vi "Lidar V5.2 RT Main.vi"() -> ()   [LabVIEW 2015]
uses:
  <vilib>/userdefined/niP2PState.ctl
  LIDAR Globals.vi
  <vilib>/Utility/error.llb/Error Cluster From Error Code.vi
  <vilib>/rvi/errors/niLvFpgaAdjustHostInterfaceError.vi
  <vilib>/rvi/interface/nirviMethod/nirviMethod.xnode
  <vilib>/rvi/interface/nirviReadWriteControl/nirviReadWriteControl.xnode
  <vilib>/rvi/errors/niLvFpgaMergeErrorWithErrorCode.vi
  <resource>/objmgr/PeerToPeerStream.rc
  <vilib>/FPGAPlugInAG/Dynamic/niLvFpga_ReadFifo_Dynamic.vi
  NiFpgaLv.dll
  <vilib>/rvi/interface/Simulation/niFpgaSimulationCallBeginRW.vi
panel:
  out "Frames":i32
  out "Slave Ref":refnum<k20>
  out "Master Ref":refnum<k20>
  out "P2P ref":refnum<k20>
  in  "Init Fpga":bool
  in  "ReadSingleFrame":bool
  out "ExitApp":bool
  out "Elements Remaining 2":u32
  in  "ReadSamples":bool
  out "Data":dbl[](graph)
  in  "stop":bool
  out "State":T1
  out "error out":errorcluster
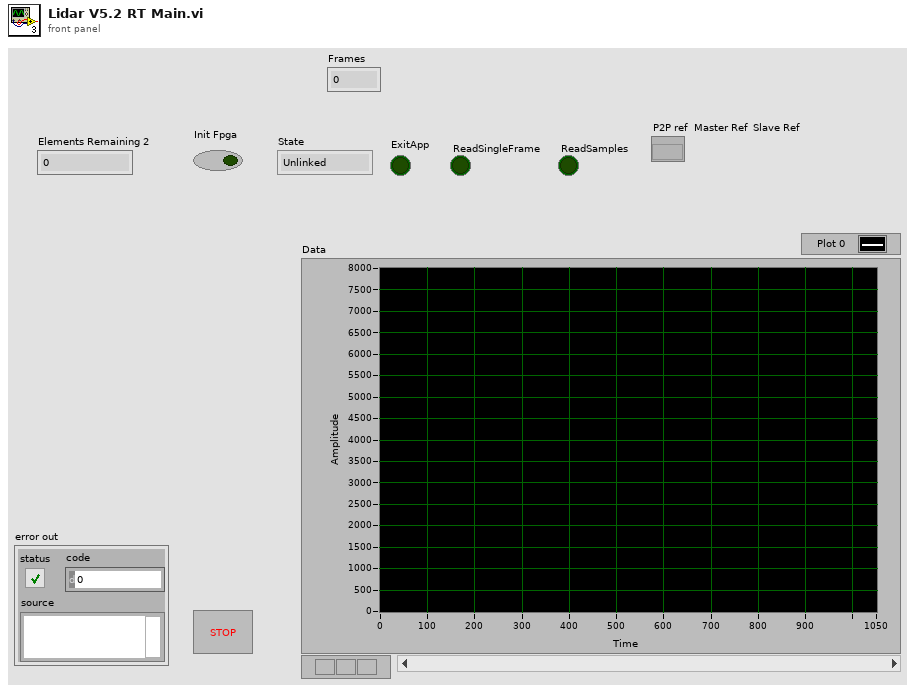
[diagram p1: front panel]
types:
  T1 = typedef "niP2PState.ctl" = enum32{"Unlinked", "Disabled", "Enabled", "Flushing"}
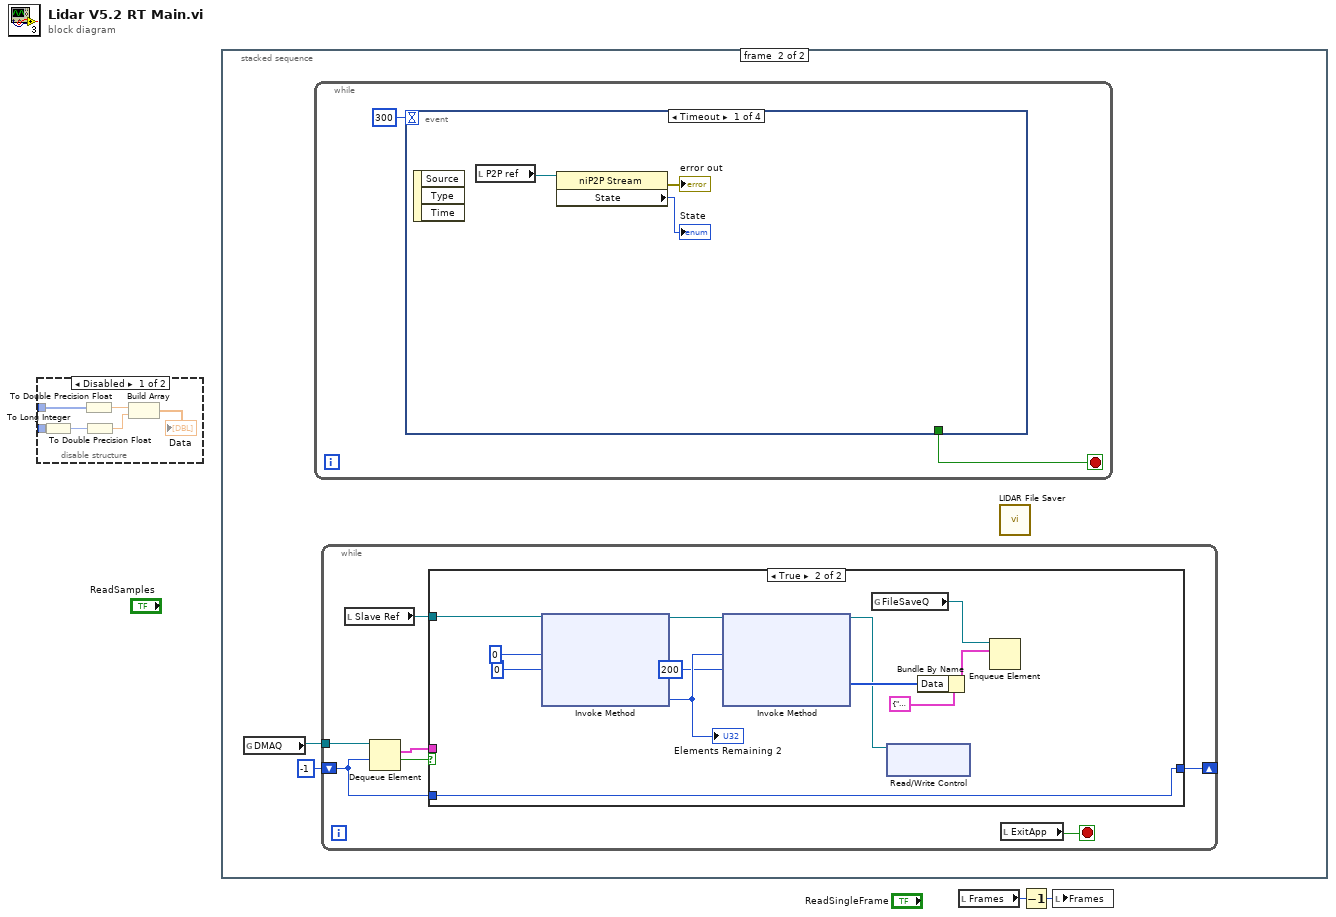
[diagram p0: block diagram]
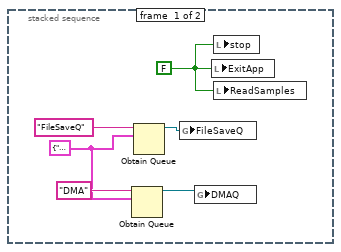
[diagram p3: hidden frame]
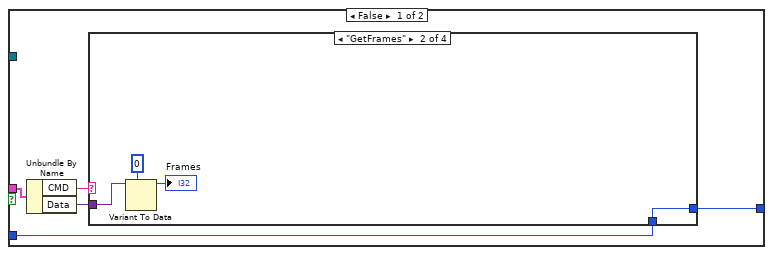
[diagram p4: hidden frame]
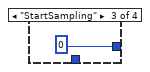
[diagram p6: hidden frame]
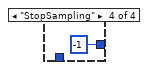
[diagram p7: hidden frame]
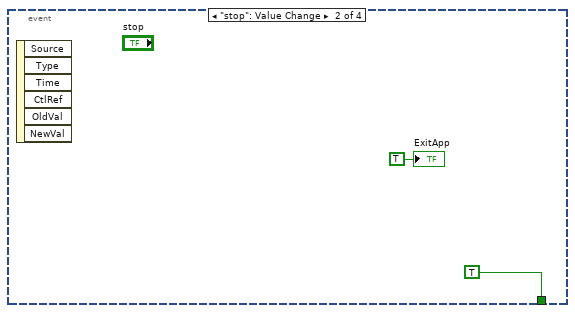
[diagram p8: hidden frame]
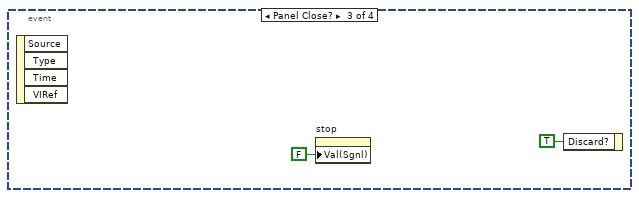
[diagram p9: hidden frame]
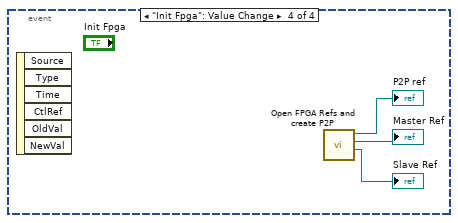
[diagram p10: hidden frame]
diagram:
  n1 = disable-structure shown="Disabled" {
    disable-tunnel: _ -> [w8 _]
    disable-tunnel: _ -> [w4 _]
    frame Disabled {
      n2 = To Long Integer(number=w8) -> (32bit integer=w7:i32)
      n3 = To Double Precision Float(number=w4) -> (double precision float=w3:dbl)
      n4 = To Double Precision Float(number=w7) -> (double precision float=w6:dbl)
      n5 = Build Array(w3, w6) -> (→"Data":dbl[])
    }
    frame Enabled {
    }
  }
  n6 = stacked-sequence {
    frame #0 {
      w12 = FALSE ("ExitApp")
      w10 = cluster{"CMD":string, "Data":variant} {"CMD"="", "Data"=variant}
      n7 = Obtain Queue(name (unnamed)="DMA", element data type=w10) -> (queue out=w9:refnum<queue>)  [unwired: 3 in, 2 out]
      n8 = Obtain Queue(name (unnamed)="FileSaveQ", element data type=w10) -> (queue out=w13:refnum<queue>)  [unwired: 3 in, 2 out]
      n9 = global write "LIDAR Globals.vi" "FileSaveQ"(w13) -> ()
      n10 = global write "LIDAR Globals.vi" "DMAQ"(w9) -> ()
      n11 = local write "ExitApp"(w12) -> ()
      n12 = local write "stop"(w12) -> ()
      n13 = local write "ReadSamples"(w12) -> ()
    }
    frame #1 {
      n14 = global read "LIDAR Globals.vi" "DMAQ"() -> (w16:refnum<queue>)
      n15 = while {
        stop <- w49 stop-if-true
        n16 = event shown="[0] Timeout" {
          selector: _ -> [_ _ _ _]
          dyn-events: _ -> [_ _ _ _]
          timeout: 300 -> [_ _ _ _]
          tunnel: [_ TRUE _ _] -> w49
          event Timeout {
            n17 = event-data() -> ()  [unwired: 1 in, 3 out]
            n18 = local read "P2P ref"() -> (w50:refnum<k20>)
            n19 = property class="niP2P Stream"(reference=w50) -> (error out=→"error out":errorcluster, "State"=→"State":T1)  [unwired: 1 in, 1 out]
          }
          event "stop": Value Change {
            n20 = event-data() -> ()  [unwired: 1 in, 6 out]
            "ExitApp" <- TRUE ("ExitApp")
          }
          event Panel Close? {
            n21 = event-data() -> ()  [unwired: 1 in, 4 out]
            n22 = property on="stop" class="Bool (strict)"("Val(Sgnl)"=FALSE ("Value (Signaling)")) -> ()  [unwired: 2 in, 2 out]
            n23 = event-data("Discard?"=TRUE) -> ()  [unwired: 1 in, 1 out]
          }
          event "Init Fpga": Value Change {
            n24 = event-data() -> ()  [unwired: 1 in, 6 out]
            n25 = call "Open FPGA Refs and create P2P.vi"() -> ("Slave Ref"=→"Slave Ref":refnum<k20>, "Master Ref"=→"Master Ref":refnum<k20>, "P2P ref"=→"P2P ref":refnum<k20>)  [unwired: 8 in, 1 out]
          }
        }
      }
      n26 = while {
        shift-right: [w18] -> _
        shift-left: -1 -> [w17]
        tunnel: w16 -> [w21]
        stop <- w23 stop-if-true
        n27 = local read "Slave Ref"() -> (w22:refnum<k20>)
        n28 = Dequeue Element(queue=w21, timeout in ms (-1)=w17) -> (element=w19:cluster{"CMD":string, "Data":variant}, timed out?=w20:bool)  [unwired: 1 in, 2 out]
        n29 = case shown="True" w20 {
          tunnel: w22 -> [_ w42]
          tunnel: w19 -> [w28 _]
          tunnel: [w26 w36] -> w18
          tunnel: w17 -> [w25 w36]
          frame False {
            n30 = Unbundle By Name(w28) -> ("CMD"=w27:string, "Data"=w24:variant)
            n31 = case shown="\"GetFrames\"" w27 {
              tunnel: [w29 w33 0 -1] -> w26
              tunnel: w25 -> [w29 w33 _ _]
              tunnel: w24 -> [_ w32 _ _]
              frame "False", Default {
              }
              frame "GetFrames" {
                n32 = Variant To Data(type=0, Variant=w32) -> (data=→"Frames":i32)  [unwired: 1 in, 1 out]
              }
              frame "StartSampling" {
              }
              frame "StopSampling" {
              }
            }
          }
          frame True {
            n33 = xnode "Invoke Method"("FPGA VI Reference In"=w42, "Number of Elements"=u32 0, "Timeout (ms)"=0) -> ("FPGA VI Reference Out"=w45:refnum<k20>, "Elements Remaining"=w47:u32)  [unwired: 1 in, 2 out]
            "Elements Remaining 2" <- w47
            n34 = xnode "Invoke Method"("FPGA VI Reference In"=w45, "Number of Elements"=w47, "Timeout (ms)"=200) -> ("FPGA VI Reference Out"=w37:refnum<k20>, "Data"=w38:u64[])  [unwired: 1 in, 2 out]
            n35 = global read "LIDAR Globals.vi" "FileSaveQ"() -> (w41:refnum<queue>)
            n36 = xnode "Read/Write Control"("FPGA VI Reference In"=w37) -> ()  [unwired: 1 in, 3 out]
            n37 = Bundle By Name(cluster=cluster{"CMD":string, "Data":variant} {"CMD"="SaveData", "Data"=variant} ("element"), "Data"=w38) -> (w39:cluster{"CMD":string, "Data":variant})
            n38 = Enqueue Element(queue=w41, element=w39) -> ()  [unwired: 2 in, 3 out]
          }
        }
        n39 = local read "ExitApp"() -> (w23:bool)
      }
      n40 = call "LIDAR File Saver.vi"() -> ()  [unwired: 12 in]
    }
  }
  n41 = local read "Frames"() -> (w1:i32)
  n42 = Decrement(x=w1) -> (x-1=w2:i32)
  n43 = local write "Frames"(w2) -> ()
